vi "Autonomous Load.vi"(0 "Number of Commands":i32, 5 "Subsystems":string[](array[string]), 7 "Commands":string[](array[string]), 9 "Inputs":string[](array[string]), 11 "error in":errorcluster) -> (4 "Queue Key":refnum<queue>, 6 "Array":i32[](array[numeric]), 8 "Autonomous Queue":refnum<queue>, 15 "errror out":errorcluster)   [LabVIEW 2019]
uses:
  Drive/Drive Control Type.ctl
  Intake/Intake Control Type.ctl
  Robot Subsystems.ctl
  Drive/Drive Notifier.ctl
  Intake/Intake Notifier.ctl
  Intake Rotation/Intake Rotation Notifier.ctl
  Intake Rotation/Intake Rotation Control Type.ctl
  Intake Rotation/Arm Enum States.ctl
  Lift/Lift Notifier.ctl
  Lift/Lift Control Type.ctl
  Lift/Lift Enum States.ctl
  RPED/RPED Notifier.ctl
  RPED/RPED Control Type.ctl
  Queue Key Data.ctl
panel:
  in  "Set Position 2":T1
  in  "Set Position":T2=enum."Climb"
  in  "Intake Rotation Control Type":T3
  in  "Lift Control Type":T4
  in  "RPED Control Type":T5
  in  "Intake Control List":T6
  out "Subsystem":string
  in  "Drive Control List":T7
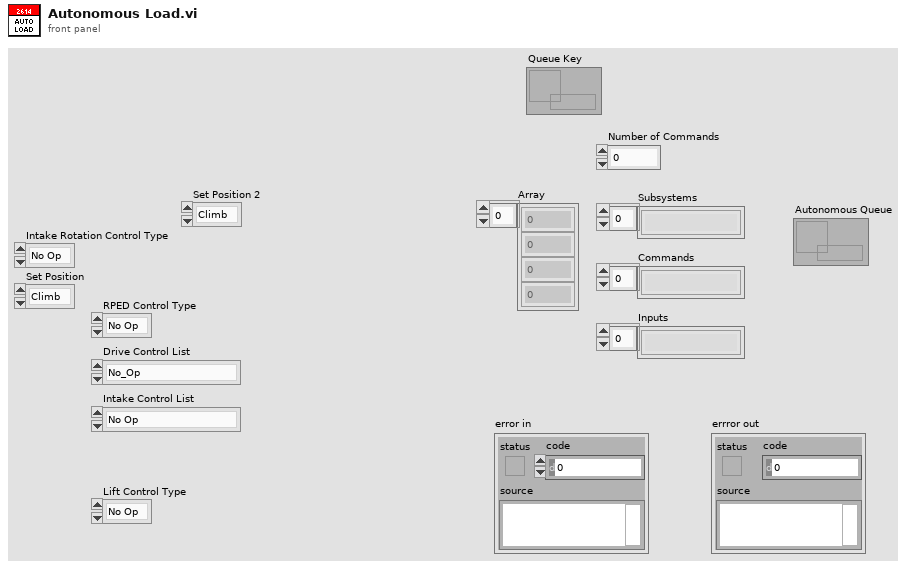
[diagram p1: front panel]
types:
  T1 = typedef "Lift Enum States.ctl" = enum16{"Climb", "Load", "Portal", "Switch", "Scale High", "Scale Mid", "Scale Low", "Exchange", "Stow", "Current Position"}
  T2 = typedef "Arm Enum States.ctl" = enum16{"Current Position", "Climb", "Load", "Portal", "Switch", "Scale High", "Scale Mid", "Scale Low", "Exchange", "Stow"}
  T3 = typedef "Intake Rotation Control Type.ctl" = enum16{"No Op", "Manual Up", "Position", "Manual Down", "PositionAuto"}
  T4 = typedef "Lift Control Type.ctl" = enum16{"No Op", "Position", "Climb Actuation", "Manual Up", "Manual Down", "PositionAuto", "Position_kP", "Position_Delay"}
  T5 = typedef "RPED Control Type.ctl" = enum16{"No Op", "Left Manual", "Right Manual", "Time", "Left", "Right", "Left_Slow", "Right_Slow", "Left_Distance", "Right_Distance"}
  T6 = typedef "Intake Control Type.ctl" = enum16{"No Op", "In", "Out", "Test Mode", "Cube_In", "Cube_Out", "State_Change"}
  T7 = typedef "Drive Control Type.ctl" = enum16{"No_Op", "Basic Drive", "Time", "Heading", "Hybrid_Turn", "RC_Speed", "Switch_Slots", "AutoTrack_Cube", "Speed Test", "Turn_Cube", "To_Cube", "Wait", "Distance_Slow", "Distance", "D_H_Delay", "Distance_Delay", "Heading_Cap", "Heading_Tight", "Cube_Heading", "Distance_Ramp"}
  T8 = typedef "Queue Key Data.ctl" = cluster{"Operation Notifier":refnum<notifier>, "Subsystem":string, "Concurrent":bool}
  T9 = typedef "Robot Subsystems.ctl" = cluster{"Drive Notifier":T10, "Intake Notifier":T11, "Intake Rotation Notifier":T12, "Lift Notifier":T13, "RPED Notifier":T14}
  T10 = typedef "Drive Notifier.ctl" = cluster{"Drive Control Type":T7, "Throttle":dbl, "Twist":dbl, "Step":i32, "High Gear":bool, "Parameter 1":dbl, "Parameter 2":dbl, "Parameter 3":dbl, "Drive Notifier":refnum<notifier>, "AutoTrack":bool}
  T11 = typedef "Intake Notifier.ctl" = cluster{"Intake Control Type":T6, "Step":i32, "In":bool, "Speed":dbl, "Out":bool, "Parameter 1":dbl, "Parameter 2":dbl, "Intake Notifier":refnum<notifier>, "Actuate Cube":bool, "Speed In":dbl, "Speed Out":dbl, "Load":bool, "Override":bool, "Exchange":bool, "Intake Open":bool}
  T12 = typedef "Intake Rotation Notifier.ctl" = cluster{"Step":i32, "Intake Rotation Control Type":T3, "Parameter 1":dbl, "Parameter 2":dbl, "Intake Rotation Notifier":refnum<notifier>, "Manual Up":bool, "Manual Down":bool, "Climb":bool, "Switch":bool, "Scale Low":bool, "Scale High":bool, "Stow":bool, "Load":bool, "Scale Mid":bool, "Exchange":bool, "Set Position":T2, "Portal":bool}
  T13 = typedef "Lift Notifier.ctl" = cluster{"Lift Control Type":T4, "Step":i32, "Set Position":T1, "Climb":bool, "Switch":bool, "Scale Low":bool, "Scale Mid":bool, "Scale High":bool, "Stow":bool, "Load":bool, "Climb Actuation":bool, "Manual Up":bool, "Manual Down":bool, "Parameter 1":dbl, "Parameter 2":dbl, "Parameter 3":dbl, "Lift Notifier":refnum<notifier>, "Exchange":bool, "Brake":bool, "Portal":bool}
  T14 = typedef "RPED Notifier.ctl" = cluster{"RPED Control Type":T5, "Step":i32, "Left Forward":bool, "Right Forward":bool, "Parameter 1":dbl, "Parameter 2":dbl, "Parameter 3":dbl, "RPED Notifier":refnum<notifier>, "Left Back":bool, "Right Back":bool, "Right":bool, "Left":bool}
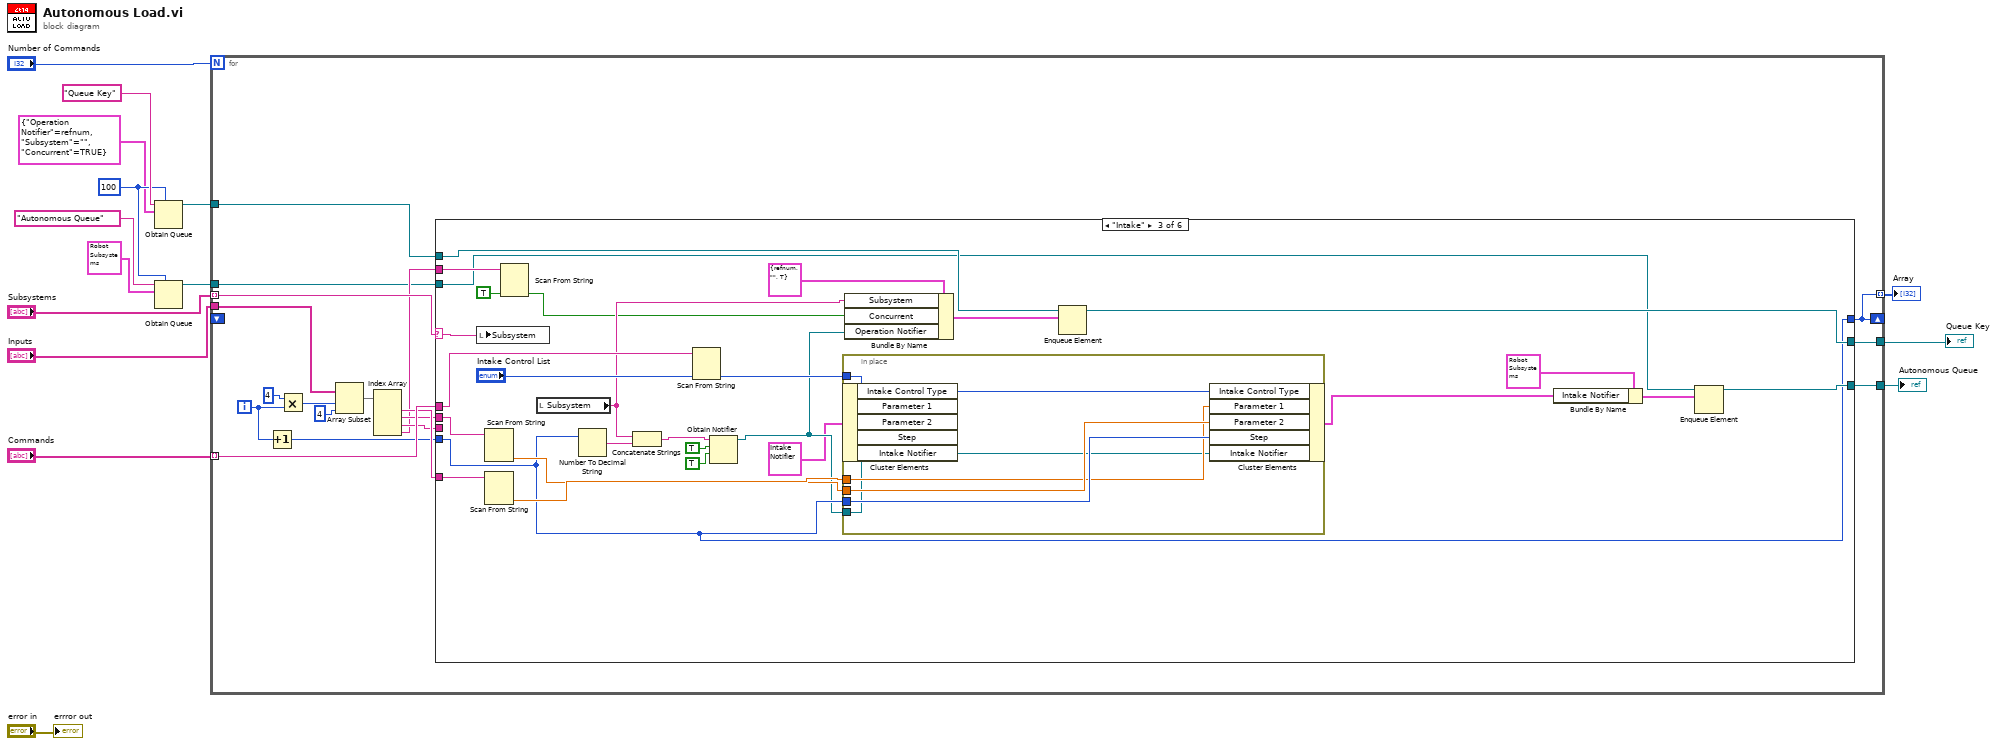
[diagram p0: block diagram]
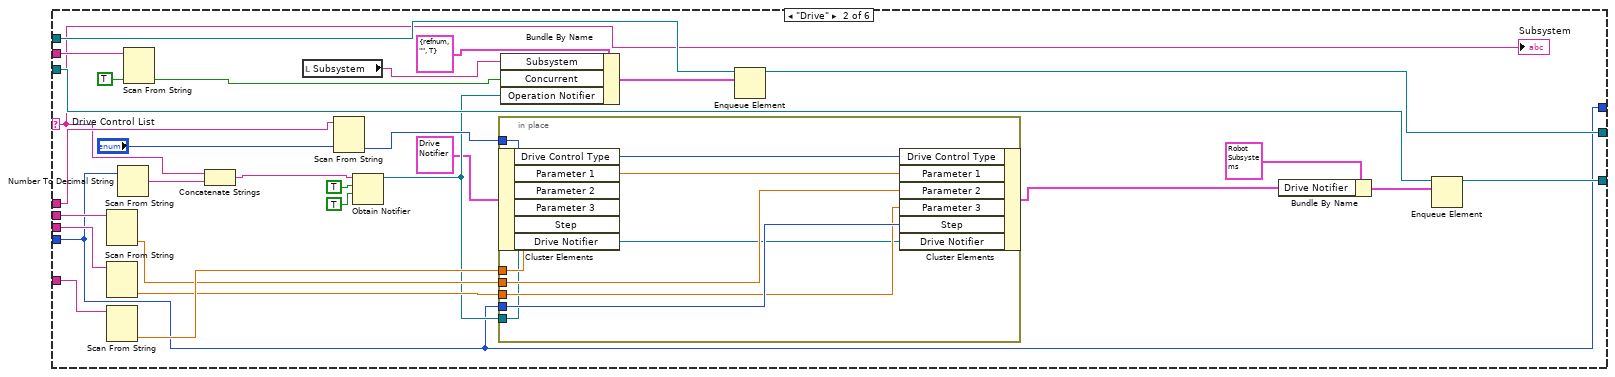
[diagram p3: hidden frame]
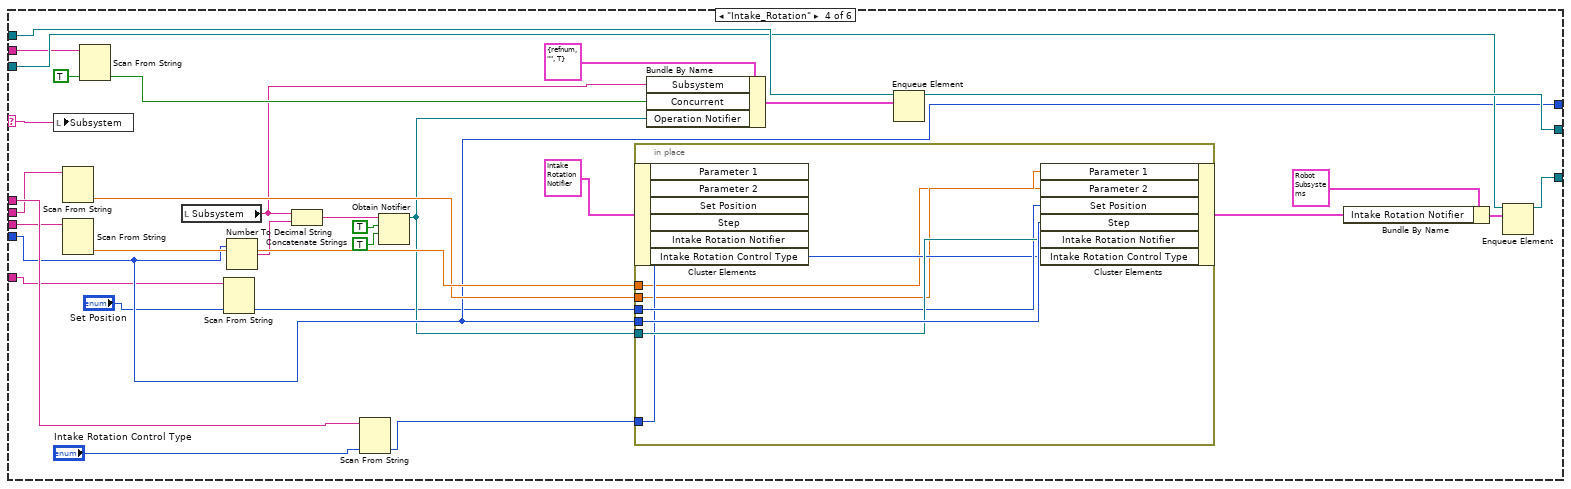
[diagram p4: hidden frame]
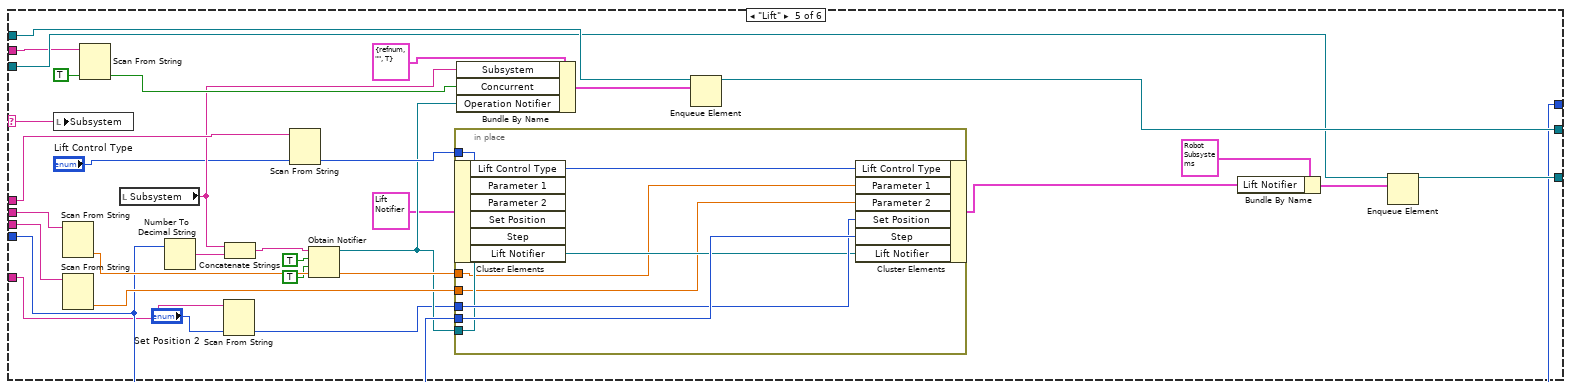
[diagram p5: hidden frame]
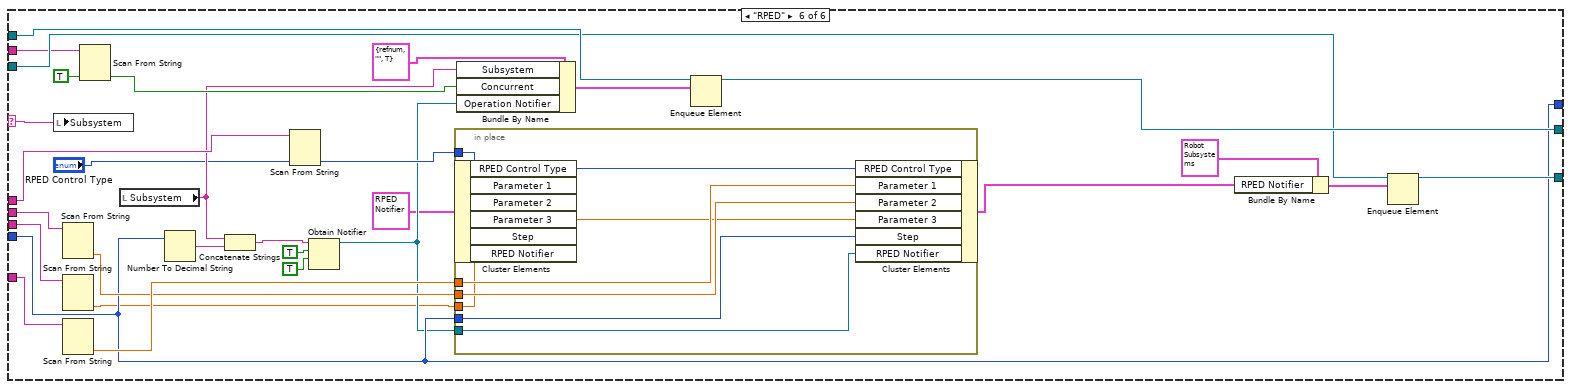
[diagram p6: hidden frame]
diagram:
  w5 = 100 ("max queue size (-1, unlimited)")
  n1 = Obtain Queue(max queue size (-1, unlimited)=w5, name (unnamed)="Queue Key", element data type=T8 {"Operation Notifier"=refnum, "Subsystem"="", "Concurrent"=TRUE} ("Queue Key Data")) -> (queue out=w13:refnum<queue>)  [unwired: 2 in, 2 out]
  n2 = Obtain Queue(max queue size (-1, unlimited)=w5, name (unnamed)="Autonomous Queue", element data type=T9 {"Drive Notifier"={"Drive Control Type"=enum."No_Op", "Throttle"=0.0, "Twist"=0.0, "Step"=0, "High Gear"=FALSE, "Parameter 1"=0.0, "Parameter 2"=0.0, "Parameter 3"=0.0, "Drive Notifier"=refnum, "AutoTrack"=FALSE}, "Intake Notifier"={"Intake Control Type"=enum."No Op", "Step"=0, "In"=FALSE, "Speed"=0.0, "Out"=FALSE, "Parameter 1"=0.0, "Parameter 2"=0.0, "Intake Notifier"=refnum, "Actuate Cube"=FALSE, "Speed In"=0.0, "Speed Out"=0.0, "Load"=FALSE, "Override"=FALSE, "Exchange"=FALSE, "Intake Open"=FALSE}, "Intake Rotation Notifier"={"Step"=0, "Intake Rotation Control Type"=enum."No Op", "Parameter 1"=0.0, "Parameter 2"=0.0, "Intake Rotation Notifier"=refnum, "Manual Up"=FALSE, "Manual Down"=FALSE, "Climb"=FALSE, "Switch"=FALSE, "Scale Low"=FALSE, "Scale High"=FALSE, "Stow"=FALSE, "Load"=FALSE, "Scale Mid"=FALSE, "Exchange"=FALSE, "Set Position"=enum."Climb", "Portal"=FALSE}, "Lift Notifier"={"Lift Control Type"=enum."No Op", "Step"=0, "Set Position"=enum."Climb", "Climb"=FALSE, "Switch"=FALSE, "Scale Low"=FALSE, "Scale Mid"=FALSE, "Scale High"=FALSE, "Stow"=FALSE, "Load"=FALSE, "Climb Actuation"=FALSE, "Manual Up"=FALSE, "Manual Down"=FALSE, "Parameter 1"=0.0, "Parameter 2"=0.0, "Parameter 3"=0.0, "Lift Notifier"=refnum, "Exchange"=FALSE, "Brake"=FALSE, "Portal"=FALSE}, "RPED Notifier"={"RPED Control Type"=enum."No Op", "Step"=0, "Left Forward"=FALSE, "Right Forward"=FALSE, "Parameter 1"=0.0, "Parameter 2"=0.0, "Parameter 3"=0.0, "RPED Notifier"=refnum, "Left Back"=FALSE, "Right Back"=FALSE, "Right"=FALSE, "Left"=FALSE}} ("Robot Subsytems")) -> (queue out=w6:refnum<queue>)  [unwired: 2 in, 2 out]
  n3 = for {
    N: "Number of Commands" -> [_]
    tunnel: w13 -> [w33]
    tunnel: "Subsystems" -> [w32] mode=indexing
    tunnel: "Commands" -> [w31] mode=indexing
    tunnel: "Inputs" -> [w26]
    tunnel: [w21] -> w2
    tunnel: w6 -> [w20]
    tunnel: [w19] -> w4
    shift-right: [w16] -> _
    shift-left: _ -> [_]
    tunnel: [w16] -> w1 mode=indexing
    i -> [w18]
    n4 = Increment(x=w18) -> (x+1=w17:i32)
    n5 = Multiply(x=4, y=w18) -> (x*y=w23:i32)
    n6 = Array Subset(array=w26, index=w23, length=4) -> (w25:string[])
    n7 = Index Array(array=w25) -> (element #1=w30:string, element #2=w29:string, element #3=w28:string, element #4=w27:string)  [unwired: 4 in]
    n8 = case shown="\"Intake\"" w32 {
      selector: w32 -> [_ w48 w94 w130 w167 w203]
      tunnel: w33 -> [w35 w63 w97 w133 w170 w206]
      tunnel: w31 -> [_ w58 w92 w129 w166 w202]
      tunnel: w30 -> [_ w57 w91 w109 w145 w201]
      tunnel: w29 -> [_ w56 w90 w128 w165 w200]
      tunnel: w28 -> [_ w55 _ w108 w144 w181]
      tunnel: w27 -> [_ w54 w89 w114 w151 w186]
      tunnel: [w36 w50 w87 w126 w163 w198] -> w19
      tunnel: [w35 w52 w86 w125 w162 w197] -> w21
      tunnel: w20 -> [w36 w51 w85 w124 w161 w196]
      tunnel: w17 -> [w34 w40 w81 w120 w157 w192]
      tunnel: [w34 w40 w81 w120 w157 w192] -> w16
      frame "No Op", Default {
      }
      frame "Drive" {
        n9 = Scan From String(input string=w56) -> (output 1=w64:dbl)  [unwired: 4 in, 3 out]
        n10 = Scan From String(input string=w55) -> (output 1=w59:dbl)  [unwired: 4 in, 3 out]
        n11 = Scan From String(input string=w57) -> (output 1=w65:dbl)  [unwired: 4 in, 3 out]
        n12 = Number To Decimal String(number=w40) -> (decimal integer string=w41:string)  [unwired: 1 in]
        n13 = Scan From String(input string=w54, default 1=TRUE) -> (output 1=w44:bool)  [unwired: 3 in, 3 out]
        n14 = Concatenate Strings(w48, w41) -> (w47:string)
        n15 = local read "Subsystem"() -> (w45:string)
        n16 = Scan From String(input string=w58, default 1="Drive Control List") -> (output 1=w66:T7)  [unwired: 3 in, 3 out]
        n17 = Obtain Notifier(name (unnamed)=w47, notification data type=TRUE, create if not found? (T)=TRUE) -> (notifier out=w43:refnum<notifier>)  [unwired: 1 in, 2 out]
        n18 = in-place {
          in-place-border: w66 -> [w72]
          in-place-border: w65 -> [w70]
          in-place-border: w64 -> [w69]
          in-place-border: w59 -> [w68]
          in-place-border: w43 -> [w67]
          in-place-border: w40 -> [w71]
          n19 = in-place-cluster #1(T10 {"Drive Control Type"=enum."No_Op", "Throttle"=0.0, "Twist"=0.0, "Step"=0, "High Gear"=FALSE, "Parameter 1"=0.0, "Parameter 2"=0.0, "Parameter 3"=0.0, "Drive Notifier"=refnum, "AutoTrack"=FALSE} ("Drive Notifier")) -> ()  [unwired: 6 out]
          n20 = in-place-cluster #1("Drive Control Type"=w72, "Parameter 1"=w70, "Parameter 2"=w69, "Parameter 3"=w68, "Step"=w71, "Drive Notifier"=w67) -> (w37:T10)
        }
        n21 = Bundle By Name(cluster=T8 {"Operation Notifier"=refnum, "Subsystem"="", "Concurrent"=TRUE} ("Queue Key Data"), "Subsystem"=w45, "Concurrent"=w44, "Operation Notifier"=w43) -> (w42:T8)
        n22 = Enqueue Element(queue=w63, element=w42) -> (queue out=w52:refnum<queue>)  [unwired: 2 in, 2 out]
        n23 = Bundle By Name(cluster=T9 {"Drive Notifier"={"Drive Control Type"=enum."No_Op", "Throttle"=0.0, "Twist"=0.0, "Step"=0, "High Gear"=FALSE, "Parameter 1"=0.0, "Parameter 2"=0.0, "Parameter 3"=0.0, "Drive Notifier"=refnum, "AutoTrack"=FALSE}, "Intake Notifier"={"Intake Control Type"=enum."No Op", "Step"=0, "In"=FALSE, "Speed"=0.0, "Out"=FALSE, "Parameter 1"=0.0, "Parameter 2"=0.0, "Intake Notifier"=refnum, "Actuate Cube"=FALSE, "Speed In"=0.0, "Speed Out"=0.0, "Load"=FALSE, "Override"=FALSE, "Exchange"=FALSE, "Intake Open"=FALSE}, "Intake Rotation Notifier"={"Step"=0, "Intake Rotation Control Type"=enum."No Op", "Parameter 1"=0.0, "Parameter 2"=0.0, "Intake Rotation Notifier"=refnum, "Manual Up"=FALSE, "Manual Down"=FALSE, "Climb"=FALSE, "Switch"=FALSE, "Scale Low"=FALSE, "Scale High"=FALSE, "Stow"=FALSE, "Load"=FALSE, "Scale Mid"=FALSE, "Exchange"=FALSE, "Set Position"=enum."Climb", "Portal"=FALSE}, "Lift Notifier"={"Lift Control Type"=enum."No Op", "Step"=0, "Set Position"=enum."Climb", "Climb"=FALSE, "Switch"=FALSE, "Scale Low"=FALSE, "Scale Mid"=FALSE, "Scale High"=FALSE, "Stow"=FALSE, "Load"=FALSE, "Climb Actuation"=FALSE, "Manual Up"=FALSE, "Manual Down"=FALSE, "Parameter 1"=0.0, "Parameter 2"=0.0, "Parameter 3"=0.0, "Lift Notifier"=refnum, "Exchange"=FALSE, "Brake"=FALSE, "Portal"=FALSE}, "RPED Notifier"={"RPED Control Type"=enum."No Op", "Step"=0, "Left Forward"=FALSE, "Right Forward"=FALSE, "Parameter 1"=0.0, "Parameter 2"=0.0, "Parameter 3"=0.0, "RPED Notifier"=refnum, "Left Back"=FALSE, "Right Back"=FALSE, "Right"=FALSE, "Left"=FALSE}} ("Robot Subsytems"), "Drive Notifier"=w37) -> (w61:T9)
        n24 = Enqueue Element(queue=w51, element=w61) -> (queue out=w50:refnum<queue>)  [unwired: 2 in, 2 out]
        "Subsystem" <- w48
      }
      frame "Intake" {
        n25 = local write "Subsystem"(w94) -> ()
        n26 = Scan From String(input string=w90) -> (output 1=w98:dbl)  [unwired: 4 in, 3 out]
        n27 = Scan From String(input string=w91) -> (output 1=w99:dbl)  [unwired: 4 in, 3 out]
        n28 = Scan From String(input string=w89, default 1=TRUE) -> (output 1=w77:bool)  [unwired: 3 in, 3 out]
        n29 = local read "Subsystem"() -> (w78:string)
        n30 = Number To Decimal String(number=w81) -> (decimal integer string=w82:string)  [unwired: 1 in]
        n31 = Concatenate Strings(w78, w82) -> (w83:string)
        n32 = Scan From String(input string=w92, default 1="Intake Control List") -> (output 1=w100:T6)  [unwired: 3 in, 3 out]
        n33 = Obtain Notifier(name (unnamed)=w83, notification data type=TRUE, create if not found? (T)=TRUE) -> (notifier out=w76:refnum<notifier>)  [unwired: 1 in, 2 out]
        n34 = in-place {
          in-place-border: w100 -> [w105]
          in-place-border: w99 -> [w102]
          in-place-border: w98 -> [w103]
          in-place-border: w76 -> [w101]
          in-place-border: w81 -> [w104]
          n35 = in-place-cluster #2(T11 {"Intake Control Type"=enum."No Op", "Step"=0, "In"=FALSE, "Speed"=0.0, "Out"=FALSE, "Parameter 1"=0.0, "Parameter 2"=0.0, "Intake Notifier"=refnum, "Actuate Cube"=FALSE, "Speed In"=0.0, "Speed Out"=0.0, "Load"=FALSE, "Override"=FALSE, "Exchange"=FALSE, "Intake Open"=FALSE} ("Intake Notifier")) -> ()  [unwired: 5 out]
          n36 = in-place-cluster #2("Intake Control Type"=w105, "Parameter 1"=w102, "Parameter 2"=w103, "Step"=w104, "Intake Notifier"=w101) -> (w73:T11)
        }
        n37 = Bundle By Name(cluster=T8 {"Operation Notifier"=refnum, "Subsystem"="", "Concurrent"=TRUE} ("Queue Key Data"), "Subsystem"=w78, "Concurrent"=w77, "Operation Notifier"=w76) -> (w79:T8)
        n38 = Enqueue Element(queue=w97, element=w79) -> (queue out=w86:refnum<queue>)  [unwired: 2 in, 2 out]
        n39 = Bundle By Name(cluster=T9 {"Drive Notifier"={"Drive Control Type"=enum."No_Op", "Throttle"=0.0, "Twist"=0.0, "Step"=0, "High Gear"=FALSE, "Parameter 1"=0.0, "Parameter 2"=0.0, "Parameter 3"=0.0, "Drive Notifier"=refnum, "AutoTrack"=FALSE}, "Intake Notifier"={"Intake Control Type"=enum."No Op", "Step"=0, "In"=FALSE, "Speed"=0.0, "Out"=FALSE, "Parameter 1"=0.0, "Parameter 2"=0.0, "Intake Notifier"=refnum, "Actuate Cube"=FALSE, "Speed In"=0.0, "Speed Out"=0.0, "Load"=FALSE, "Override"=FALSE, "Exchange"=FALSE, "Intake Open"=FALSE}, "Intake Rotation Notifier"={"Step"=0, "Intake Rotation Control Type"=enum."No Op", "Parameter 1"=0.0, "Parameter 2"=0.0, "Intake Rotation Notifier"=refnum, "Manual Up"=FALSE, "Manual Down"=FALSE, "Climb"=FALSE, "Switch"=FALSE, "Scale Low"=FALSE, "Scale High"=FALSE, "Stow"=FALSE, "Load"=FALSE, "Scale Mid"=FALSE, "Exchange"=FALSE, "Set Position"=enum."Climb", "Portal"=FALSE}, "Lift Notifier"={"Lift Control Type"=enum."No Op", "Step"=0, "Set Position"=enum."Climb", "Climb"=FALSE, "Switch"=FALSE, "Scale Low"=FALSE, "Scale Mid"=FALSE, "Scale High"=FALSE, "Stow"=FALSE, "Load"=FALSE, "Climb Actuation"=FALSE, "Manual Up"=FALSE, "Manual Down"=FALSE, "Parameter 1"=0.0, "Parameter 2"=0.0, "Parameter 3"=0.0, "Lift Notifier"=refnum, "Exchange"=FALSE, "Brake"=FALSE, "Portal"=FALSE}, "RPED Notifier"={"RPED Control Type"=enum."No Op", "Step"=0, "Left Forward"=FALSE, "Right Forward"=FALSE, "Parameter 1"=0.0, "Parameter 2"=0.0, "Parameter 3"=0.0, "RPED Notifier"=refnum, "Left Back"=FALSE, "Right Back"=FALSE, "Right"=FALSE, "Left"=FALSE}} ("Robot Subsytems"), "Intake Notifier"=w73) -> (w96:T9)
        n40 = Enqueue Element(queue=w85, element=w96) -> (queue out=w87:refnum<queue>)  [unwired: 2 in, 2 out]
      }
      frame "Intake_Rotation" {
        n41 = local write "Subsystem"(w130) -> ()
        n42 = Scan From String(input string=w128) -> (output 1=w134:dbl)  [unwired: 4 in, 3 out]
        n43 = Scan From String(input string=w108) -> (output 1=w135:dbl)  [unwired: 4 in, 3 out]
        n44 = Scan From String(input string=w114, default 1=TRUE) -> (output 1=w116:bool)  [unwired: 3 in, 3 out]
        n45 = local read "Subsystem"() -> (w115:string)
        n46 = Scan From String(input string=w109, default 1="Set Position") -> (output 1=w110:T2)  [unwired: 3 in, 3 out]
        n47 = Number To Decimal String(number=w120) -> (decimal integer string=w121:string)  [unwired: 1 in]
        n48 = Concatenate Strings(w115, w121) -> (w122:string)
        n49 = Scan From String(input string=w129, default 1="Intake Rotation Control Type") -> (output 1=w136:T3)  [unwired: 3 in, 3 out]
        n50 = Obtain Notifier(name (unnamed)=w122, notification data type=TRUE, create if not found? (T)=TRUE) -> (notifier out=w117:refnum<notifier>)  [unwired: 1 in, 2 out]
        n51 = in-place {
          in-place-border: w136 -> [w139]
          in-place-border: w135 -> [w137]
          in-place-border: w134 -> [w138]
          in-place-border: w117 -> [w141]
          in-place-border: w120 -> [w142]
          in-place-border: w110 -> [w140]
          n52 = in-place-cluster #3(T12 {"Step"=0, "Intake Rotation Control Type"=enum."No Op", "Parameter 1"=0.0, "Parameter 2"=0.0, "Intake Rotation Notifier"=refnum, "Manual Up"=FALSE, "Manual Down"=FALSE, "Climb"=FALSE, "Switch"=FALSE, "Scale Low"=FALSE, "Scale High"=FALSE, "Stow"=FALSE, "Load"=FALSE, "Scale Mid"=FALSE, "Exchange"=FALSE, "Set Position"=enum."Climb", "Portal"=FALSE} ("Intake Rotation Notifier")) -> ()  [unwired: 6 out]
          n53 = in-place-cluster #3("Parameter 1"=w138, "Parameter 2"=w137, "Set Position"=w140, "Step"=w142, "Intake Rotation Notifier"=w141, "Intake Rotation Control Type"=w139) -> (w111:T12)
        }
        n54 = Bundle By Name(cluster=T8 {"Operation Notifier"=refnum, "Subsystem"="", "Concurrent"=TRUE} ("Queue Key Data"), "Subsystem"=w115, "Concurrent"=w116, "Operation Notifier"=w117) -> (w118:T8)
        n55 = Enqueue Element(queue=w133, element=w118) -> (queue out=w125:refnum<queue>)  [unwired: 2 in, 2 out]
        n56 = Bundle By Name(cluster=T9 {"Drive Notifier"={"Drive Control Type"=enum."No_Op", "Throttle"=0.0, "Twist"=0.0, "Step"=0, "High Gear"=FALSE, "Parameter 1"=0.0, "Parameter 2"=0.0, "Parameter 3"=0.0, "Drive Notifier"=refnum, "AutoTrack"=FALSE}, "Intake Notifier"={"Intake Control Type"=enum."No Op", "Step"=0, "In"=FALSE, "Speed"=0.0, "Out"=FALSE, "Parameter 1"=0.0, "Parameter 2"=0.0, "Intake Notifier"=refnum, "Actuate Cube"=FALSE, "Speed In"=0.0, "Speed Out"=0.0, "Load"=FALSE, "Override"=FALSE, "Exchange"=FALSE, "Intake Open"=FALSE}, "Intake Rotation Notifier"={"Step"=0, "Intake Rotation Control Type"=enum."No Op", "Parameter 1"=0.0, "Parameter 2"=0.0, "Intake Rotation Notifier"=refnum, "Manual Up"=FALSE, "Manual Down"=FALSE, "Climb"=FALSE, "Switch"=FALSE, "Scale Low"=FALSE, "Scale High"=FALSE, "Stow"=FALSE, "Load"=FALSE, "Scale Mid"=FALSE, "Exchange"=FALSE, "Set Position"=enum."Climb", "Portal"=FALSE}, "Lift Notifier"={"Lift Control Type"=enum."No Op", "Step"=0, "Set Position"=enum."Climb", "Climb"=FALSE, "Switch"=FALSE, "Scale Low"=FALSE, "Scale Mid"=FALSE, "Scale High"=FALSE, "Stow"=FALSE, "Load"=FALSE, "Climb Actuation"=FALSE, "Manual Up"=FALSE, "Manual Down"=FALSE, "Parameter 1"=0.0, "Parameter 2"=0.0, "Parameter 3"=0.0, "Lift Notifier"=refnum, "Exchange"=FALSE, "Brake"=FALSE, "Portal"=FALSE}, "RPED Notifier"={"RPED Control Type"=enum."No Op", "Step"=0, "Left Forward"=FALSE, "Right Forward"=FALSE, "Parameter 1"=0.0, "Parameter 2"=0.0, "Parameter 3"=0.0, "RPED Notifier"=refnum, "Left Back"=FALSE, "Right Back"=FALSE, "Right"=FALSE, "Left"=FALSE}} ("Robot Subsytems"), "Intake Rotation Notifier"=w111) -> (w132:T9)
        n57 = Enqueue Element(queue=w124, element=w132) -> (queue out=w126:refnum<queue>)  [unwired: 2 in, 2 out]
      }
      frame "Lift" {
        n58 = local write "Subsystem"(w167) -> ()
        n59 = Scan From String(input string=w165) -> (output 1=w171:dbl)  [unwired: 4 in, 3 out]
        n60 = Scan From String(input string=w144) -> (output 1=w172:dbl)  [unwired: 4 in, 3 out]
        n61 = Scan From String(input string=w151, default 1=TRUE) -> (output 1=w153:bool)  [unwired: 3 in, 3 out]
        n62 = local read "Subsystem"() -> (w152:string)
        n63 = Number To Decimal String(number=w157) -> (decimal integer string=w158:string)  [unwired: 1 in]
        n64 = Scan From String(input string=w145, default 1="Set Position 2") -> (output 1=w147:T1)  [unwired: 3 in, 3 out]
        n65 = Concatenate Strings(w152, w158) -> (w159:string)
        n66 = Scan From String(input string=w166, default 1="Lift Control Type") -> (output 1=w173:T4)  [unwired: 3 in, 3 out]
        n67 = Obtain Notifier(name (unnamed)=w159, notification data type=TRUE, create if not found? (T)=TRUE) -> (notifier out=w154:refnum<notifier>)  [unwired: 1 in, 2 out]
        n68 = in-place {
          in-place-border: w173 -> [w179]
          in-place-border: w172 -> [w175]
          in-place-border: w171 -> [w174]
          in-place-border: w154 -> [w176]
          in-place-border: w157 -> [w178]
          in-place-border: w147 -> [w177]
          n69 = in-place-cluster #4(T13 {"Lift Control Type"=enum."No Op", "Step"=0, "Set Position"=enum."Climb", "Climb"=FALSE, "Switch"=FALSE, "Scale Low"=FALSE, "Scale Mid"=FALSE, "Scale High"=FALSE, "Stow"=FALSE, "Load"=FALSE, "Climb Actuation"=FALSE, "Manual Up"=FALSE, "Manual Down"=FALSE, "Parameter 1"=0.0, "Parameter 2"=0.0, "Parameter 3"=0.0, "Lift Notifier"=refnum, "Exchange"=FALSE, "Brake"=FALSE, "Portal"=FALSE} ("Lift Notifier")) -> ()  [unwired: 6 out]
          n70 = in-place-cluster #4("Lift Control Type"=w179, "Parameter 1"=w174, "Parameter 2"=w175, "Set Position"=w177, "Step"=w178, "Lift Notifier"=w176) -> (w146:T13)
        }
        n71 = Bundle By Name(cluster=T8 {"Operation Notifier"=refnum, "Subsystem"="", "Concurrent"=TRUE} ("Queue Key Data"), "Subsystem"=w152, "Concurrent"=w153, "Operation Notifier"=w154) -> (w155:T8)
        n72 = Enqueue Element(queue=w170, element=w155) -> (queue out=w162:refnum<queue>)  [unwired: 2 in, 2 out]
        n73 = Bundle By Name(cluster=T9 {"Drive Notifier"={"Drive Control Type"=enum."No_Op", "Throttle"=0.0, "Twist"=0.0, "Step"=0, "High Gear"=FALSE, "Parameter 1"=0.0, "Parameter 2"=0.0, "Parameter 3"=0.0, "Drive Notifier"=refnum, "AutoTrack"=FALSE}, "Intake Notifier"={"Intake Control Type"=enum."No Op", "Step"=0, "In"=FALSE, "Speed"=0.0, "Out"=FALSE, "Parameter 1"=0.0, "Parameter 2"=0.0, "Intake Notifier"=refnum, "Actuate Cube"=FALSE, "Speed In"=0.0, "Speed Out"=0.0, "Load"=FALSE, "Override"=FALSE, "Exchange"=FALSE, "Intake Open"=FALSE}, "Intake Rotation Notifier"={"Step"=0, "Intake Rotation Control Type"=enum."No Op", "Parameter 1"=0.0, "Parameter 2"=0.0, "Intake Rotation Notifier"=refnum, "Manual Up"=FALSE, "Manual Down"=FALSE, "Climb"=FALSE, "Switch"=FALSE, "Scale Low"=FALSE, "Scale High"=FALSE, "Stow"=FALSE, "Load"=FALSE, "Scale Mid"=FALSE, "Exchange"=FALSE, "Set Position"=enum."Climb", "Portal"=FALSE}, "Lift Notifier"={"Lift Control Type"=enum."No Op", "Step"=0, "Set Position"=enum."Climb", "Climb"=FALSE, "Switch"=FALSE, "Scale Low"=FALSE, "Scale Mid"=FALSE, "Scale High"=FALSE, "Stow"=FALSE, "Load"=FALSE, "Climb Actuation"=FALSE, "Manual Up"=FALSE, "Manual Down"=FALSE, "Parameter 1"=0.0, "Parameter 2"=0.0, "Parameter 3"=0.0, "Lift Notifier"=refnum, "Exchange"=FALSE, "Brake"=FALSE, "Portal"=FALSE}, "RPED Notifier"={"RPED Control Type"=enum."No Op", "Step"=0, "Left Forward"=FALSE, "Right Forward"=FALSE, "Parameter 1"=0.0, "Parameter 2"=0.0, "Parameter 3"=0.0, "RPED Notifier"=refnum, "Left Back"=FALSE, "Right Back"=FALSE, "Right"=FALSE, "Left"=FALSE}} ("Robot Subsytems"), "Lift Notifier"=w146) -> (w169:T9)
        n74 = Enqueue Element(queue=w161, element=w169) -> (queue out=w163:refnum<queue>)  [unwired: 2 in, 2 out]
      }
      frame "RPED" {
        n75 = local write "Subsystem"(w203) -> ()
        n76 = Scan From String(input string=w200) -> (output 1=w207:dbl)  [unwired: 4 in, 3 out]
        n77 = Scan From String(input string=w181) -> (output 1=w180:dbl)  [unwired: 4 in, 3 out]
        n78 = Scan From String(input string=w201) -> (output 1=w208:dbl)  [unwired: 4 in, 3 out]
        n79 = Scan From String(input string=w186, default 1=TRUE) -> (output 1=w188:bool)  [unwired: 3 in, 3 out]
        n80 = local read "Subsystem"() -> (w187:string)
        n81 = Number To Decimal String(number=w192) -> (decimal integer string=w193:string)  [unwired: 1 in]
        n82 = Concatenate Strings(w187, w193) -> (w194:string)
        n83 = Scan From String(input string=w202, default 1="RPED Control Type") -> (output 1=w209:T5)  [unwired: 3 in, 3 out]
        n84 = Obtain Notifier(name (unnamed)=w194, notification data type=TRUE, create if not found? (T)=TRUE) -> (notifier out=w189:refnum<notifier>)  [unwired: 1 in, 2 out]
        n85 = in-place {
          in-place-border: w209 -> [w215]
          in-place-border: w208 -> [w214]
          in-place-border: w207 -> [w213]
          in-place-border: w189 -> [w212]
          in-place-border: w192 -> [w211]
          in-place-border: w180 -> [w210]
          n86 = in-place-cluster #5(T14 {"RPED Control Type"=enum."No Op", "Step"=0, "Left Forward"=FALSE, "Right Forward"=FALSE, "Parameter 1"=0.0, "Parameter 2"=0.0, "Parameter 3"=0.0, "RPED Notifier"=refnum, "Left Back"=FALSE, "Right Back"=FALSE, "Right"=FALSE, "Left"=FALSE} ("RPED Notifier")) -> ()  [unwired: 6 out]
          n87 = in-place-cluster #5("RPED Control Type"=w215, "Parameter 1"=w214, "Parameter 2"=w213, "Parameter 3"=w210, "Step"=w211, "RPED Notifier"=w212) -> (w182:T14)
        }
        n88 = Bundle By Name(cluster=T8 {"Operation Notifier"=refnum, "Subsystem"="", "Concurrent"=TRUE} ("Queue Key Data"), "Subsystem"=w187, "Concurrent"=w188, "Operation Notifier"=w189) -> (w190:T8)
        n89 = Enqueue Element(queue=w206, element=w190) -> (queue out=w197:refnum<queue>)  [unwired: 2 in, 2 out]
        n90 = Bundle By Name(cluster=T9 {"Drive Notifier"={"Drive Control Type"=enum."No_Op", "Throttle"=0.0, "Twist"=0.0, "Step"=0, "High Gear"=FALSE, "Parameter 1"=0.0, "Parameter 2"=0.0, "Parameter 3"=0.0, "Drive Notifier"=refnum, "AutoTrack"=FALSE}, "Intake Notifier"={"Intake Control Type"=enum."No Op", "Step"=0, "In"=FALSE, "Speed"=0.0, "Out"=FALSE, "Parameter 1"=0.0, "Parameter 2"=0.0, "Intake Notifier"=refnum, "Actuate Cube"=FALSE, "Speed In"=0.0, "Speed Out"=0.0, "Load"=FALSE, "Override"=FALSE, "Exchange"=FALSE, "Intake Open"=FALSE}, "Intake Rotation Notifier"={"Step"=0, "Intake Rotation Control Type"=enum."No Op", "Parameter 1"=0.0, "Parameter 2"=0.0, "Intake Rotation Notifier"=refnum, "Manual Up"=FALSE, "Manual Down"=FALSE, "Climb"=FALSE, "Switch"=FALSE, "Scale Low"=FALSE, "Scale High"=FALSE, "Stow"=FALSE, "Load"=FALSE, "Scale Mid"=FALSE, "Exchange"=FALSE, "Set Position"=enum."Climb", "Portal"=FALSE}, "Lift Notifier"={"Lift Control Type"=enum."No Op", "Step"=0, "Set Position"=enum."Climb", "Climb"=FALSE, "Switch"=FALSE, "Scale Low"=FALSE, "Scale Mid"=FALSE, "Scale High"=FALSE, "Stow"=FALSE, "Load"=FALSE, "Climb Actuation"=FALSE, "Manual Up"=FALSE, "Manual Down"=FALSE, "Parameter 1"=0.0, "Parameter 2"=0.0, "Parameter 3"=0.0, "Lift Notifier"=refnum, "Exchange"=FALSE, "Brake"=FALSE, "Portal"=FALSE}, "RPED Notifier"={"RPED Control Type"=enum."No Op", "Step"=0, "Left Forward"=FALSE, "Right Forward"=FALSE, "Parameter 1"=0.0, "Parameter 2"=0.0, "Parameter 3"=0.0, "RPED Notifier"=refnum, "Left Back"=FALSE, "Right Back"=FALSE, "Right"=FALSE, "Left"=FALSE}} ("Robot Subsytems"), "RPED Notifier"=w182) -> (w205:T9)
        n91 = Enqueue Element(queue=w196, element=w205) -> (queue out=w198:refnum<queue>)  [unwired: 2 in, 2 out]
      }
    }
  }
  "Autonomous Queue" <- w4
  "Queue Key" <- w2
  "Array" <- w1
  "errror out" <- "error in"
